vi "U16To16Bits.vi"(11 "Nombre à convertir":u16) -> (3 "Array of bits":u16[](array[numeric]))   [LabVIEW 2014]
panel:
  out "power of 2":u16[](array[numeric])
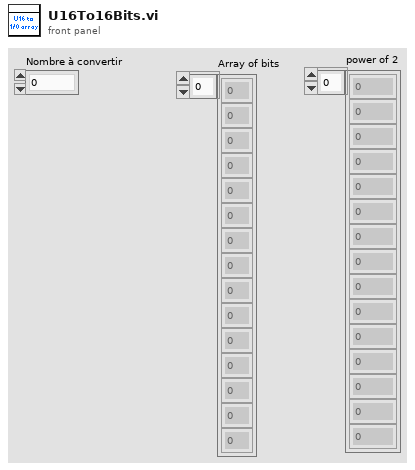
[diagram p1: front panel]
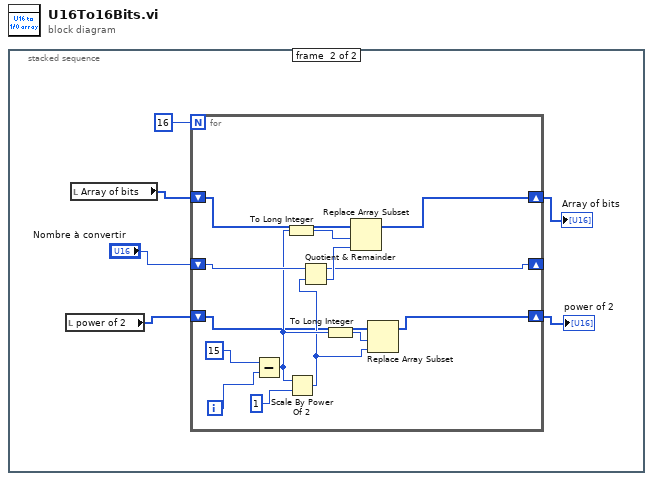
[diagram p0: block diagram]
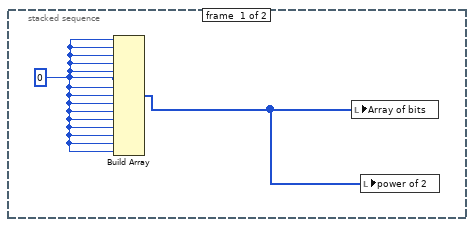
[diagram p2: hidden frame]
diagram:
  n1 = stacked-sequence {
    frame #0 {
      w2 = u16 0
      n2 = Build Array(w2, w2, w2, w2, w2, w2, w2, w2, w2, w2, w2, w2, w2, w2, w2) -> (w1:u16[])
      n3 = local write "Array of bits"(w1) -> ()
      n4 = local write "power of 2"(w1) -> ()
    }
    frame #1 {
      n5 = local read "power of 2"() -> (w4:u16[])
      n6 = local read "Array of bits"() -> (w6:u16[])
      n7 = for {
        N: 16 -> [_]
        shift-right: [w18] -> _
        shift-left: "Nombre à convertir" -> [w21]
        shift-right: [w16] -> w5
        shift-left: w6 -> [w17]
        shift-right: [w12] -> w3
        shift-left: w4 -> [w13]
        i -> [w9]
        n8 = Subtract(x=u16 15, y=w9) -> (x-y=w15:i32)
        n9 = To Long Integer(number=w15) -> (32bit integer=w11:i32)
        n10 = Scale By Power Of 2(n=w15, x=u16 1) -> (x*2^n=w14:u16)
        n11 = Quotient & Remainder(x=w21, y=w14) -> (x-y*floor(x/y)=w18:u16, floor(x/y)=w19:u16)
        n12 = To Long Integer(number=w15) -> (32bit integer=w10:i32)
        n13 = Replace Array Subset(array=w17, new element=w19, index=w11) -> (w16:u16[])
        n14 = Replace Array Subset(array=w13, new element=w14, index=w10) -> (w12:u16[])
      }
      "Array of bits" <- w5
      "power of 2" <- w3
    }
  }
